vi "init.vi"(8 "error in (no error)":errorcluster, 11 "Encoder in":refnum<class "Encoder.lvclass">) -> (0 "error out":errorcluster, 3 "Encoder out":refnum<class "Encoder.lvclass">)   [LabVIEW 2013, in "Encoder.lvclass"]
uses:
  Encoder.lvclass
  Configuration/Encoder.ctl
  Encoder.lvclass/Encoder.ctl
  ConfigurationThisComponent/ConfigurationThisComponent.lvclass
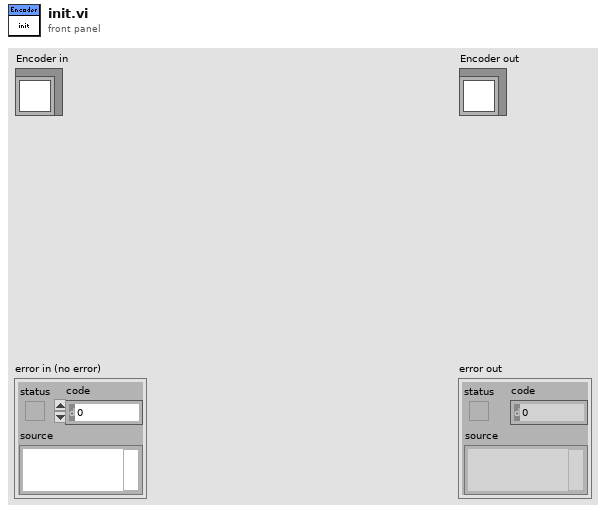
[diagram p1: front panel]
types:
  T1 = typedef "Encoder.ctl" = cluster{"Distance Per Count":dbl[unit]}
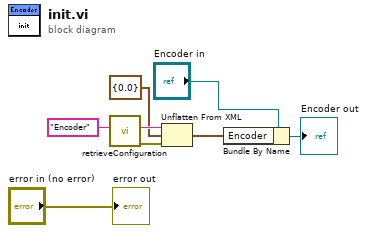
[diagram p0: block diagram]
diagram:
  n1 = call "retrieveConfiguration.vi"("configName"="Encoder") -> ("error out"=w5:errorcluster, "xmlConfig"=w6:string)  [unwired: 8 in, 1 out]
  n2 = Unflatten From XML(xml string=w6, type=T1 {"Distance Per Count"=0.0} ("Encoder"), error in (no error)=w5) -> (value=w1:T1)  [unwired: 1 out]
  n3 = Bundle By Name(cluster="Encoder in", "Encoder"=w1) -> (→"Encoder out":refnum<class "Encoder.lvclass">)
  "error out" <- "error in (no error)"
